vi "Rings In A Cluster - No Type Defs.vi"(10 "String":string, 11 "Cluster":T1={"Numeric"=0.0, "Inner Cluster - Level 1"={"String"="", "Enum"=enum."CCCC", "Boolean"=FALSE, "Cluster"={"Numeric"=0.0, "String"="", "Text Ring"=2233.0}, "Array Of Enums"=[enum."Enum Value - 1", enum."Enum Value - 3", enum."Enum Value - 4"]}} {"Inner Cluster - Level 1"."Cluster"."Text Ring" items=["Text Ring Value 1", "Text Ring Value 2", "Text Ring Value 3", "Text Ring Value 4", "Text Ring Value 5"]}) -> ()   [LabVIEW 2012]
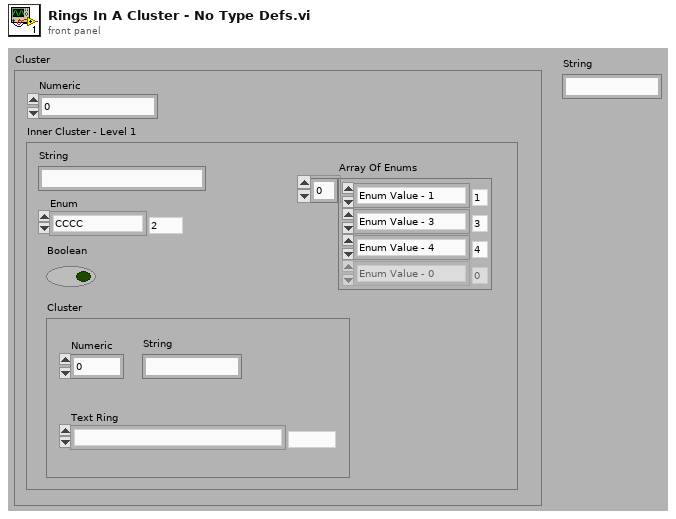
[diagram p1: front panel]
types:
  T1 = cluster{"Numeric":dbl, "Inner Cluster - Level 1":cluster{"String":string, "Enum":enum8{"AAA", "BBB", "CCCC", "DDDD", "EEEE"}, "Boolean":bool, "Cluster":cluster{"Numeric":dbl, "String":string, "Text Ring":ext}, "Array Of Enums":enum16{"Enum Value - 0", "Enum Value - 1", "Enum Value - 2", "Enum Value - 3", "Enum Value - 4"}[]}}
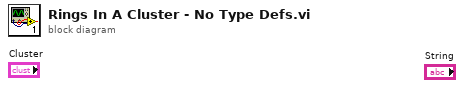
[diagram p0: block diagram]
diagram:
